vi "Convert Variant To Section.vi"(8 "error in":errorcluster, 11 "Section Variant":variant) -> (0 "error out":errorcluster, 3 "Section Ref out":refnum<data-value>)   [LabVIEW 2024, in "Config File Parser.lvlib" / "Section.lvclass"]
uses:
  Section.lvclass
  Section.lvclass/Section.ctl
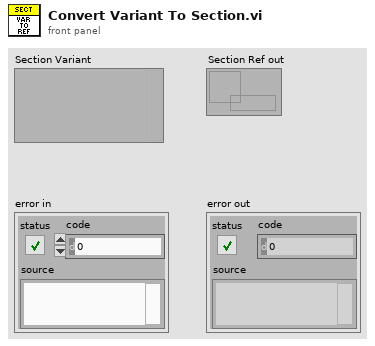
[diagram p1: front panel]
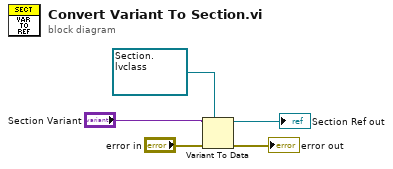
[diagram p0: block diagram]
diagram:
  n1 = Variant To Data(error in="error in", type=refnum<data-value> refnum ("Section Ref constant"), Variant="Section Variant") -> (data=→"Section Ref out":refnum<data-value>, error out=→"error out":errorcluster)
